vi "Calculate_Row_Time.vi"(0 "Multi Run Row":T1 {"Carrier_2 Q (l/min)" format="%#.2f"; "Row Duration (mins)" format="%#.1f"; "Row No" min=0; "Trace Gas Concentration (%)" min=0.0 format="%#_4f"; "Carrier_1 Q (l/min)" format="%#.4f"; "Start X" format="%#.2f"; "Start Y" format="%#.2f"; "Start Z" format="%#.2f"; "End X" format="%#.2f"; "End Y" format="%#.2f"; "End Z" format="%#.2f"; "Tunnel Speed" format="%#.2f"; "Averaging time (mins)" min=0.0 format="%#.2f"}, 1 "Row Start Time (Sec Since 1904)":dbl) -> (2 "Fixed Time (Sec)":dbl format="%.2f", 3 "Scalable Time (Sec)":dbl format="%.2f", 4 "waitTime (Sec)":dbl format="%.2f")   [LabVIEW 2020]
uses:
  Traverse_cluster.ctl
  Spacing.ctl
  Controls/Multi_run_mode.ctl
  Globals/Preference_global.vi
  Globals/Extra_Commands_Global.vi
panel:
  # "X           Y          Z"
  # "Start"
  # "End"
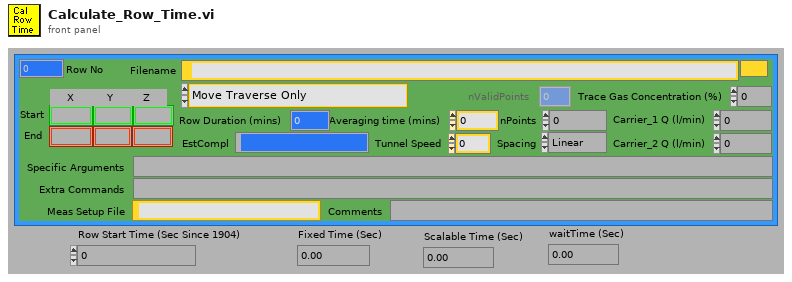
[diagram p1: front panel]
types:
  T1 = typedef "Traverse_cluster.ctl" = cluster{"Start X":sgl, "Start Y":sgl, "Start Z":sgl, "End X":sgl, "End Y":sgl, "End Z":sgl, "nPoints":i32, "Spacing":T2, "Filename":path, "Tunnel Speed":dbl, "Averaging time (mins)":dbl, "Extra Commands":string, "Carrier_1 Q (l/min)":dbl, "Carrier_2 Q (l/min)":dbl, "Trace Gas Concentration (%)":dbl, "Specific Arguments":string, "Comments":string, "Row No":i32, "Row Type Selector":T3, "EstCompl":string, "Row Duration (mins)":dbl, "nValidPoints":i32, "Meas Setup File":string}
  T2 = typedef "Spacing.ctl" = enum16{"Linear", "Log", "Gauss", "Specified", "N/A"}
  T3 = typedef "Multi_run_mode.ctl" = enum16{"Move Traverse Only", "Set Tunnel Speed Only", "Set Source Only", "Set Measurement Conditions", "Single Measurement", "Vertical Profile", "Lateral Profile", "Longitudinal Profile", "Multi-Axis Profile", "Explore Volume", "Auto Calibrate", "Meas Fast FID Bkgnd", "Check Beam Power", "Scanning Valve Measurement", "Run VI Named:", "Set ADAM Ch", "Wait (minutes)", "Send Message", "Synchronize With:", "Fall Back to this Row", "Turn Off Row Repeating", "Traverse 3D Volume", "Blank Row", "Jump to Fall Back Row"}
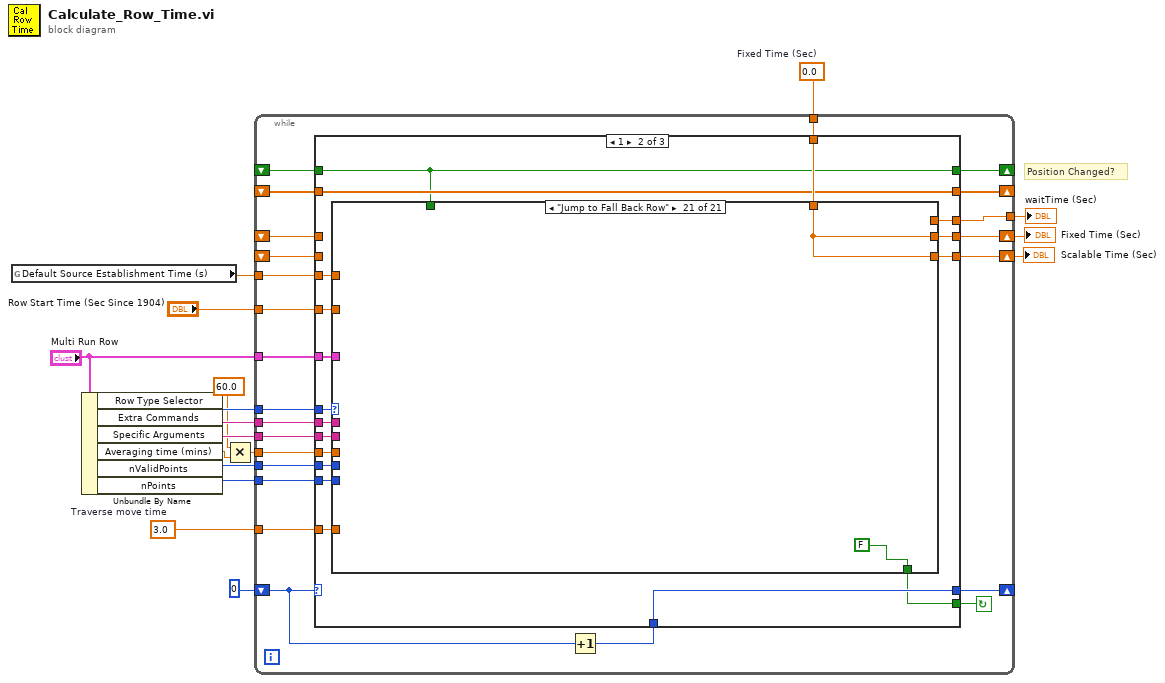
[diagram p0: block diagram]
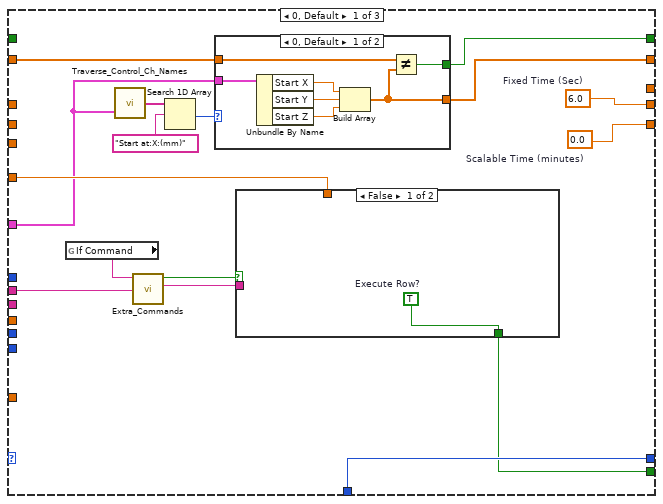
[diagram p2: hidden frame]
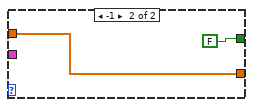
[diagram p3: hidden frame]
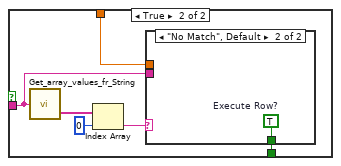
[diagram p4: hidden frame]
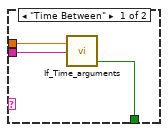
[diagram p5: hidden frame]
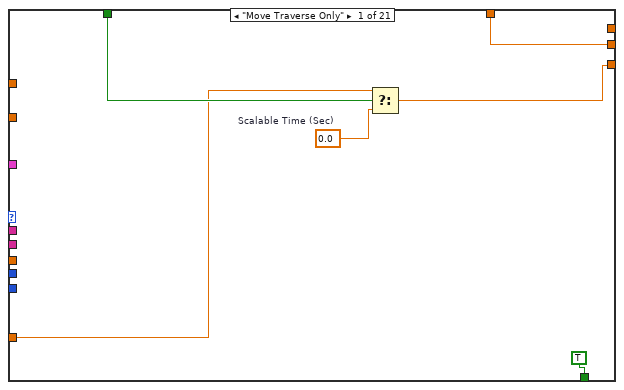
[diagram p6: hidden frame]
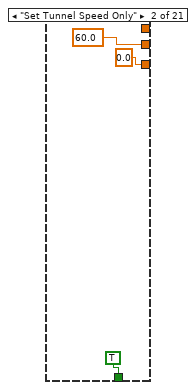
[diagram p7: hidden frame]
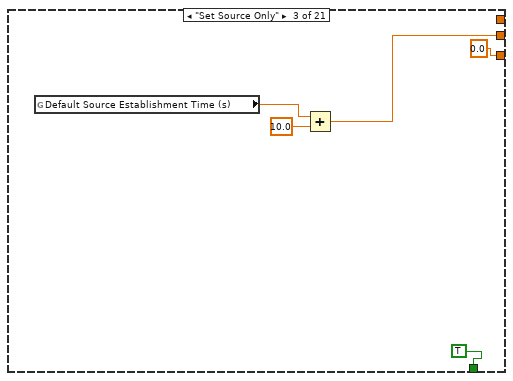
[diagram p8: hidden frame]
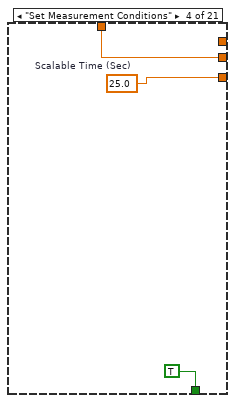
[diagram p9: hidden frame]
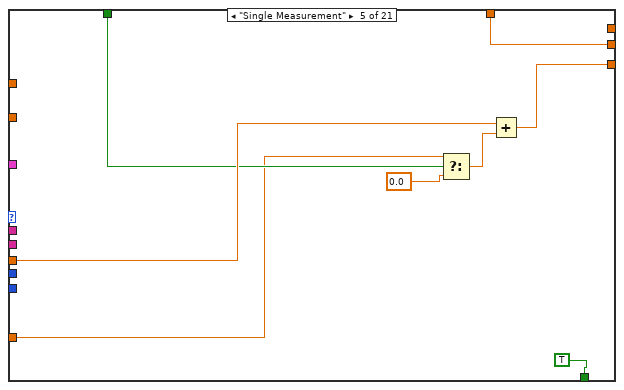
[diagram p10: hidden frame]
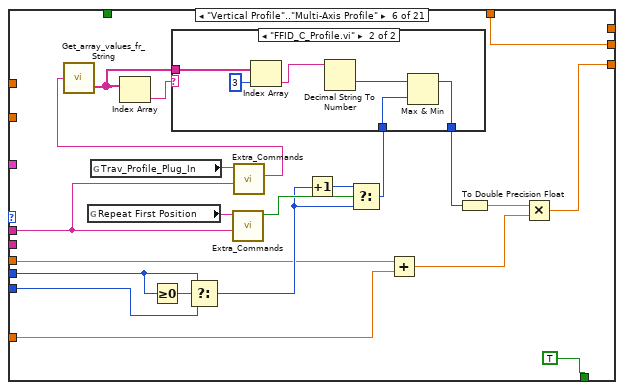
[diagram p11: hidden frame]
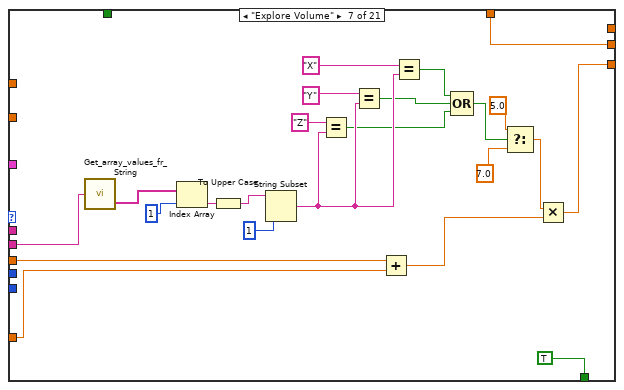
[diagram p13: hidden frame]
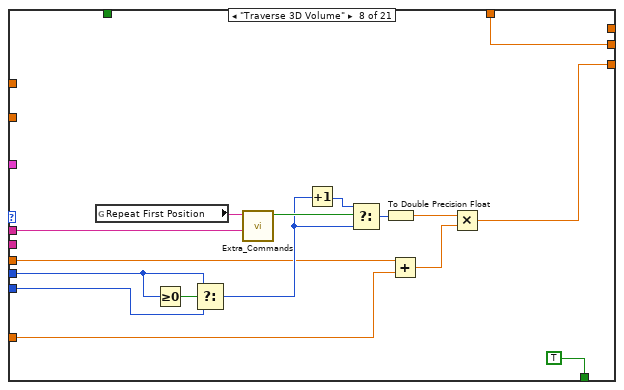
[diagram p14: hidden frame]
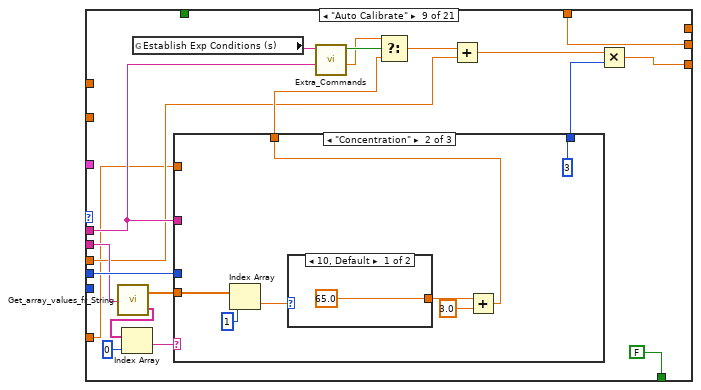
[diagram p15: hidden frame]
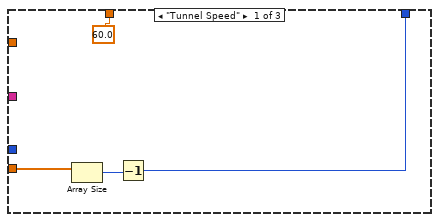
[diagram p16: hidden frame]
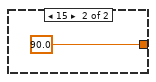
[diagram p17: hidden frame]
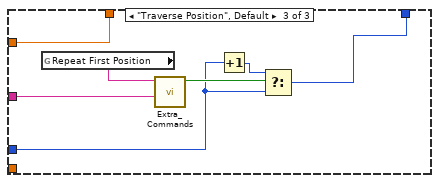
[diagram p18: hidden frame]
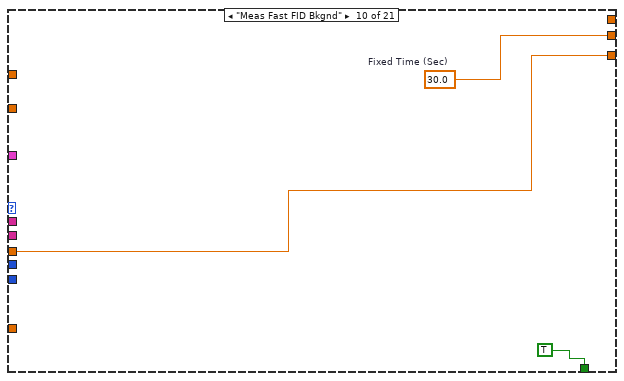
[diagram p19: hidden frame]
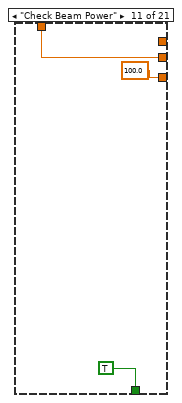
[diagram p20: hidden frame]
diagram:
  w1 = 3.0  # Traverse move time
  w6 = 0.0  # Fixed Time (Sec)
  # "Position Changed?"
  n1 = global read "Preference_global.vi" "Default Source Establishment Time (s)"() -> (w3:dbl)
  n2 = Unbundle By Name("Multi Run Row") -> ("Row Type Selector"=w12:T3, "Extra Commands"=w16:string, "Specific Arguments"=w10:string, "Averaging time (mins)"=w9:dbl, "nValidPoints"=w11:i32, "nPoints"=w5:i32)
  n3 = Multiply(x=60.0, y=w9) -> (x*y=w7:dbl)
  n4 = while {
    tunnel: w6 -> [w27]
    tunnel: w10 -> [w30]
    tunnel: w11 -> [w31]
    tunnel: w7 -> [w32]
    tunnel: w12 -> [w33]
    tunnel: "Row Start Time (Sec Since 1904)" -> [w36]
    tunnel: w16 -> [w37]
    shift-left: _ -> [w29]
    shift-right: [w34] -> w14
    shift-left: _ -> [w28]
    shift-right: [w35] -> w13
    shift-left: 0 -> [w40]
    shift-right: [w38] -> _
    tunnel: w5 -> [w26]
    tunnel: "Multi Run Row" -> [w25]
    shift-right: [w24] -> _
    shift-left: _ -> [w23]
    shift-right: [w22] -> _
    shift-left: _ -> [w21]
    tunnel: w3 -> [w20]
    tunnel: [w19] -> w2
    tunnel: w1 -> [w18]
    stop <- w41 continue-if-true
    n5 = Increment(x=w40) -> (x+1=w39:i32)
    n6 = case shown="1" w40 {
      tunnel: [w52 w85 FALSE ("Execute Row?")] -> w41
      tunnel: w39 -> [w57 w94 w275]
      tunnel: [w57 w94 w275] -> w38
      tunnel: w37 -> [w53 w90 w280]
      tunnel: w36 -> [w51 w87 _]
      tunnel: [w50 w93 w277] -> w35
      tunnel: [w49 w92 w282] -> w34
      tunnel: w33 -> [_ w95 _]
      tunnel: w32 -> [_ w91 _]
      tunnel: w31 -> [_ w89 _]
      tunnel: w30 -> [_ w88 _]
      tunnel: w29 -> [_ _ w282]
      tunnel: w28 -> [_ _ w278]
      tunnel: w27 -> [_ w86 _]
      tunnel: w26 -> [_ w84 _]
      tunnel: w25 -> [w45 w80 _]
      tunnel: [w44 w83 w272] -> w24
      tunnel: w23 -> [w43 w83 w272]
      tunnel: [w42 w82 w273] -> w22
      tunnel: w21 -> [_ w82 w273]
      tunnel: w20 -> [_ w81 _]
      tunnel: [_ w79 _] -> w19
      tunnel: w18 -> [_ w78 _]
      frame 0, Default {
        w50 = 6.0  # Fixed Time (Sec)
        w49 = 0.0  # Scalable Time (minutes)
        n7 = global read "Extra_Commands_Global.vi" "If Command"() -> (w55:string)
        n8 = call "Traverse_Control_Ch_Names.vi"("Traverse line"=w45) -> ("Channel names"=w48:string[])  [unwired: 1 in]
        n9 = call "Extra_Commands.vi"("String to Search"=w53, "Command"=w55) -> ("String Value"=w54:string, "Command Found"=w56:bool)  [unwired: 1 in, 3 out]
        n10 = Search 1D Array(1D array=w48, element="Start at:X:(mm)" ("Label for value")) -> (index of element=w46:i32)  [unwired: 1 out]
        n11 = case shown="0, Default" w46 {
          tunnel: w45 -> [w64 _]
          tunnel: [w60 w66] -> w44
          tunnel: w43 -> [w59 w66]
          tunnel: [w58 FALSE] -> w42
          frame 0, Default {
            n12 = Unbundle By Name(w64) -> ("Start X"=w63:sgl, "Start Y"=w62:sgl, "Start Z"=w61:sgl)
            n13 = Build Array(w63, w62, w61) -> (w60:sgl[])
            n14 = Not Equal?(x=w59, y=w60) -> (x != y?=w58:bool)
          }
          frame -1 {
          }
        }
        n15 = case shown="False" w56 {
          tunnel: w54 -> [_ w70]
          tunnel: [w67 w69] -> w52
          tunnel: w51 -> [_ w68]
          frame False {
            w67 = TRUE  # Execute Row?
          }
          frame True {
            n16 = call "Get_array_values_fr_String.vi"("String Value"=w70) -> ("String array"=w72:string[])  [unwired: 1 out]
            n17 = Index Array(array=w72, index=0 ("Index")) -> (element=w71:string)
            n18 = case shown="\"No Match\", Default" w71 {
              tunnel: w70 -> [w76 _]
              tunnel: [w75 w77] -> w69
              tunnel: w68 -> [w74 _]
              frame "Time Between" {
                n19 = call "If_Time_arguments.vi"("seconds since 1Jan1904"=w74, "String Value"=w76) -> ("Execute Row?"=w75:bool)  [unwired: 2 out]
              }
              frame "No Match", Default {
                w77 = TRUE  # Execute Row?
              }
            }
          }
        }
      }
      frame 1 {
        n20 = case shown="\"Jump to Fall Back Row\"" w95 {
          tunnel: [w101 60.0 ("Scalable Time (Sec)") w106 w111 w120 w136 w170 w180 w196 w229 w231 w237 w238 w242 w249 w257 w260 w263 w266 w269 w271] -> w93
          tunnel: [w97 0.0 0.0 w110 w115 w138 w171 w183 w197 w228 100.0 w233 w240 w241 w255 w258 w261 w264 w267 w269 w271] -> w92
          tunnel: w91 -> [_ _ _ _ w117 w130 w168 w174 w191 w228 _ w234 _ _ _ _ _ _ _ _ _]
          tunnel: w90 -> [_ _ _ _ _ w123 _ w186 w200 _ _ _ _ _ _ _ _ _ _ _ _]
          tunnel: w89 -> [_ _ _ _ _ w133 _ w176 w206 _ _ _ _ _ _ _ _ _ _ _ _]
          tunnel: w88 -> [_ _ _ _ _ _ w161 _ w203 _ _ _ _ w246 w254 _ _ _ _ _ _]
          tunnel: w87 -> [_ _ _ _ _ _ _ _ _ _ _ _ _ _ w253 _ _ _ _ _ _]
          tunnel: w86 -> [w101 _ _ w111 w120 w136 w170 w180 w196 _ w231 w237 w238 _ _ w257 w260 w263 w266 w269 w271]
          tunnel: [TRUE TRUE TRUE TRUE TRUE TRUE TRUE TRUE FALSE TRUE TRUE TRUE TRUE TRUE FALSE TRUE TRUE FALSE FALSE FALSE FALSE] -> w85
          tunnel: w84 -> [_ _ _ _ _ w132 _ w177 _ _ _ _ _ _ _ _ _ _ _ _ _]
          tunnel: w82 -> [w99 _ _ _ w114 _ _ _ _ _ _ _ _ _ _ _ _ _ _ _ _]
          tunnel: w81 -> [_ _ _ _ _ _ _ _ _ _ _ _ _ _ _ _ _ _ _ _ _]
          tunnel: w80 -> [_ _ _ _ _ _ _ _ _ _ _ _ _ w243 _ _ _ _ _ _ _]
          tunnel: [_ _ _ _ _ _ _ _ _ _ _ _ _ _ w249 _ _ _ _ _ _] -> w79
          tunnel: w78 -> [w96 _ _ _ w113 w121 w149 w172 w188 _ _ _ _ _ _ _ _ _ _ _ _]
          frame "Move Traverse Only" {
            w98 = 0.0  # Scalable Time (Sec)
            n21 = Select(t=w96, s=w99, f=w98) -> (s? t:f=w97:dbl)
          }
          frame "Set Tunnel Speed Only" {
          }
          frame "Set Source Only" {
            n22 = global read "Preference_global.vi" "Default Source Establishment Time (s)"() -> (w108:dbl)
            n23 = Add(x=w108, y=10.0) -> (x+y=w106:dbl)
          }
          frame "Set Measurement Conditions" {
            w110 = 25.0  # Scalable Time (Sec)
          }
          frame "Single Measurement" {
            n24 = Select(t=w113, s=w114, f=0.0 ("Scalable Time (Sec)")) -> (s? t:f=w116:dbl)
            n25 = Add(x=w117, y=w116) -> (x+y=w115:dbl)
          }
          frame "Vertical Profile".."Multi-Axis Profile" {
            n26 = global read "Extra_Commands_Global.vi" "Repeat First Position"() -> (w141:string)
            n27 = global read "Extra_Commands_Global.vi" "Trav_Profile_Plug_In"() -> (w124:string)
            n28 = Greater Or Equal To 0?(x=w133) -> (x >= 0?=w134:bool)
            n29 = Select(t=w133, s=w134, f=w132) -> (s? t:f=w131:i32)
            n30 = call "Extra_Commands.vi"("String to Search"=w123, "Command"=w141) -> ("Command Found"=w140:bool)  [unwired: 1 in, 4 out]
            n31 = call "Extra_Commands.vi"("String to Search"=w123, "Command"=w124) -> ("String Value"=w122:string)  [unwired: 1 in, 4 out]
            n32 = call "Get_array_values_fr_String.vi"("String Value"=w122) -> ("String array"=w127:string[])  [unwired: 1 out]
            n33 = Index Array(array=w127) -> (element=w128:string)  [unwired: 1 in]
            n34 = Increment(x=w131) -> (x+1=w139:i32)
            n35 = Select(t=w139, s=w140, f=w131) -> (s? t:f=w126:i32)
            n36 = case shown="\"FFID_C_Profile.vi\"" w128 {
              tunnel: w127 -> [_ w148]
              tunnel: w126 -> [w142 w144]
              tunnel: [w142 w143] -> w125
              frame Default {
              }
              frame "FFID_C_Profile.vi" {
                n37 = Index Array(array=w148, index=3) -> (element=w146:string)
                n38 = Decimal String To Number(string=w146) -> (number=w145:i32)  [unwired: 2 in, 1 out]
                n39 = Max & Min(x=w145, y=w144) -> (max(x,y)=w143:i32)  [unwired: 1 out]
              }
            }
            n40 = Add(x=w130, y=w121) -> (x+y=w129:dbl)
            n41 = To Double Precision Float(number=w125) -> (double precision float=w137:dbl)
            n42 = Multiply(x=w137, y=w129) -> (x*y=w138:dbl)
          }
          frame "Explore Volume" {
            n43 = call "Get_array_values_fr_String.vi"("String Value"=w161) -> ("String array"=w166:string[])  [unwired: 1 out]
            n44 = Index Array(array=w166, index=1) -> (element=w164:string)
            n45 = To Upper Case(1:w164) -> (0:w163:string)
            n46 = String Subset(string=w163, length (rest)=1 ("length (rest)")) -> (substring=w157:string)  [unwired: 1 in]
            n47 = Equal?(x="Z", y=w157) -> (x = y?=w154:bool)
            n48 = Equal?(x="Y", y=w157) -> (x = y?=w155:bool)
            n49 = Add(x=w168, y=w149) -> (x+y=w167:dbl)
            n50 = Equal?(x="X", y=w157) -> (x = y?=w156:bool)
            n51 = Compound Arithmetic op=OR(w156, w155, w154) -> (w152:bool)
            n52 = Select(t=5.0, s=w152, f=7.0 ("x")) -> (s? t:f=w151:dbl)
            n53 = Multiply(x=w151, y=w167) -> (x*y=w171:dbl)
          }
          frame "Traverse 3D Volume" {
            n54 = global read "Extra_Commands_Global.vi" "Repeat First Position"() -> (w187:string)
            n55 = Greater Or Equal To 0?(x=w176) -> (x >= 0?=w178:bool)
            n56 = Select(t=w176, s=w178, f=w177) -> (s? t:f=w175:i32)
            n57 = call "Extra_Commands.vi"("String to Search"=w186, "Command"=w187) -> ("Command Found"=w185:bool)  [unwired: 1 in, 4 out]
            n58 = Increment(x=w175) -> (x+1=w184:i32)
            n59 = Select(t=w184, s=w185, f=w175) -> (s? t:f=w182:i32)
            n60 = To Double Precision Float(number=w182) -> (double precision float=w181:dbl)
            n61 = Add(x=w174, y=w172) -> (x+y=w173:dbl)
            n62 = Multiply(x=w181, y=w173) -> (x*y=w183:dbl)
          }
          frame "Auto Calibrate" {
            n63 = call "Get_array_values_fr_String.vi"("String Value"=w203) -> ("Numeric Array"=w199:dbl[], "String array"=w205:string[])
            n64 = Index Array(array=w205, index=0 ("Index")) -> (element=w202:string)
            n65 = global read "Extra_Commands_Global.vi" "Establish Exp Conditions (s)"() -> (w201:string)
            n66 = case shown="\"Concentration\"" w202 {
              tunnel: w200 -> [_ _ w225]
              tunnel: w206 -> [_ _ w223]
              tunnel: [w208 3 ("No. of pts.") w221] -> w198
              tunnel: w199 -> [w210 w215 _]
              tunnel: [60.0 w211 w220] -> w193
              tunnel: w188 -> [_ _ w220]
              frame "Tunnel Speed" {
                n67 = Array Size(array=w210) -> (size(s)=w209:i32)
                n68 = Decrement(x=w209) -> (x-1=w208:i32)
              }
              frame "Concentration" {
                n69 = Index Array(array=w215, index=1) -> (element=w214:dbl)
                n70 = case shown="10, Default" w214 {
                  tunnel: [65.0 ("Seconds to wait") 90.0 ("Seconds to wait")] -> w213
                  frame 10, Default {
                  }
                  frame 15 {
                  }
                }
                n71 = Add(x=w213, y=3.0) -> (x+y=w211:dbl)
              }
              frame "Traverse Position", Default {
                n72 = global read "Extra_Commands_Global.vi" "Repeat First Position"() -> (w226:string)
                n73 = call "Extra_Commands.vi"("String to Search"=w225, "Command"=w226) -> ("Command Found"=w224:bool)  [unwired: 1 in, 4 out]
                n74 = Increment(x=w223) -> (x+1=w222:i32)
                n75 = Select(t=w222, s=w224, f=w223) -> (s? t:f=w221:i32)
              }
            }
            n76 = call "Extra_Commands.vi"("String to Search"=w200, "Command"=w201) -> ("Numeric Value"=w194:dbl, "Command Found"=w195:bool)  [unwired: 1 in, 3 out]
            n77 = Select(t=w194, s=w195, f=w193) -> (s? t:f=w192:dbl)
            n78 = Add(x=w192, y=w191) -> (x+y=w190:dbl)
            n79 = Multiply(x=w190, y=w198) -> (x*y=w197:dbl)
          }
          frame "Meas Fast FID Bkgnd" {
            w229 = 30.0  # Fixed Time (Sec)
          }
          frame "Check Beam Power" {
          }
          frame "Scanning Valve Measurement" {
            n80 = Add(x=w234, y=5.0 ("Scalable Time (Sec)")) -> (x+y=w233:dbl)
          }
          frame "Set ADAM Ch" {
            w240 = 1.0  # Scalable Time (Sec)
          }
          frame "Run VI Named:" {
            n81 = Match Pattern(string=w246, regular expression=";") -> (before substring=w245:string)  [unwired: 4 out]
            n82 = call <vilib>:"Trim Whitespace.vi"("string"=w245) -> ("trimmed string"=w244:string)  [unwired: 1 in]
            n83 = call "Run_VI_Named_specific.vi"("Run VI Named String"=w244, "Multi Run Row"=w243) -> ("Scalable Time (Sec)"=w241:dbl, "Fixed Time (Sec)"=w242:dbl)  [unwired: 1 in, 7 out]
          }
          frame "Wait (minutes)" {
            w255 = 0.0  # Scalable Time (Sec)
            n84 = call "Wait_Case_Arg.vi"("Specific Argument"=w254, "seconds since 1Jan1904"=w253) -> ("Minutes To Wait"=w252:dbl)  [unwired: 4 out]
            n85 = Multiply(x=w252, y=60.0) -> (x*y=w249:dbl)
          }
          frame "Send Message" {
            w258 = 1.0  # Scalable Time (Sec)
          }
          frame "Synchronize With:" {
            w261 = 30.0  # Scalable Time (Sec)
          }
          frame "Fall Back to this Row" {
            w264 = 1.0  # Scalable Time (Sec)
          }
          frame "Turn Off Row Repeating" {
            w267 = 1.0  # Scalable Time (Sec)
          }
          frame "Blank Row" {
          }
          frame "Jump to Fall Back Row" {
          }
        }
      }
      frame 2 {
        n86 = global read "Extra_Commands_Global.vi" "Establish Exp Conditions (s)"() -> (w281:string)
        n87 = call "Extra_Commands.vi"("String to Search"=w280, "Command"=w281) -> ("Numeric Value"=w279:dbl, "Command Found"=w276:bool)  [unwired: 1 in, 3 out]
        n88 = case shown="True" w276 {
          tunnel: w279 -> [_ w284]
          tunnel: w278 -> [w283 w286]
          tunnel: [w283 w285] -> w277
          frame False {
          }
          frame True {
            n89 = Add(x=w286, y=w284) -> (x+y=w285:dbl)
          }
        }
      }
    }
  }
  "Fixed Time (Sec)" <- w13
  "Scalable Time (Sec)" <- w14
  "waitTime (Sec)" <- w2
